vi "PTSAutoDailyEric.vi"() -> ()   [LabVIEW 2012]
uses:
  <vilib>/Utility/NIReport.llb/NI_report.lvclass
  <vilib>/addons/database/Connection.llb/DB Tools Open Connec (Path).vi
  <vilib>/addons/database/Connection.llb/Conn Execute.vi
  <vilib>/addons/database/Recordset.llb/Rec Fetch Recordset Data (R).vi
  <vilib>/addons/database/Recordset.llb/Rec Destroy - Connection.vi
  <vilib>/Utility/NIReport.llb/Append Text Table to Report (wrap).vi
  <vilib>/addons/database/_DB Variant To Data/Database Variant To Data.xnode
  <vilib>/addons/database/NI_Database_API.lvlib
  <vilib>/Utility/NIReport.llb/Excel/NI_Excel.lvclass
  <vilib>/addons/_office/NI_ReportGenerationToolkit.lvlib
panel:
  in  "Report Template":path=path "O:/Monitor/Report/PTSDailyReport.xls"
  in  "Table Control":string[][](table)
  out "error out 4":errorcluster
  out "error out":errorcluster
  out "appended array":string[](array[string])
  out "recordset data":variant[][](array[variant])
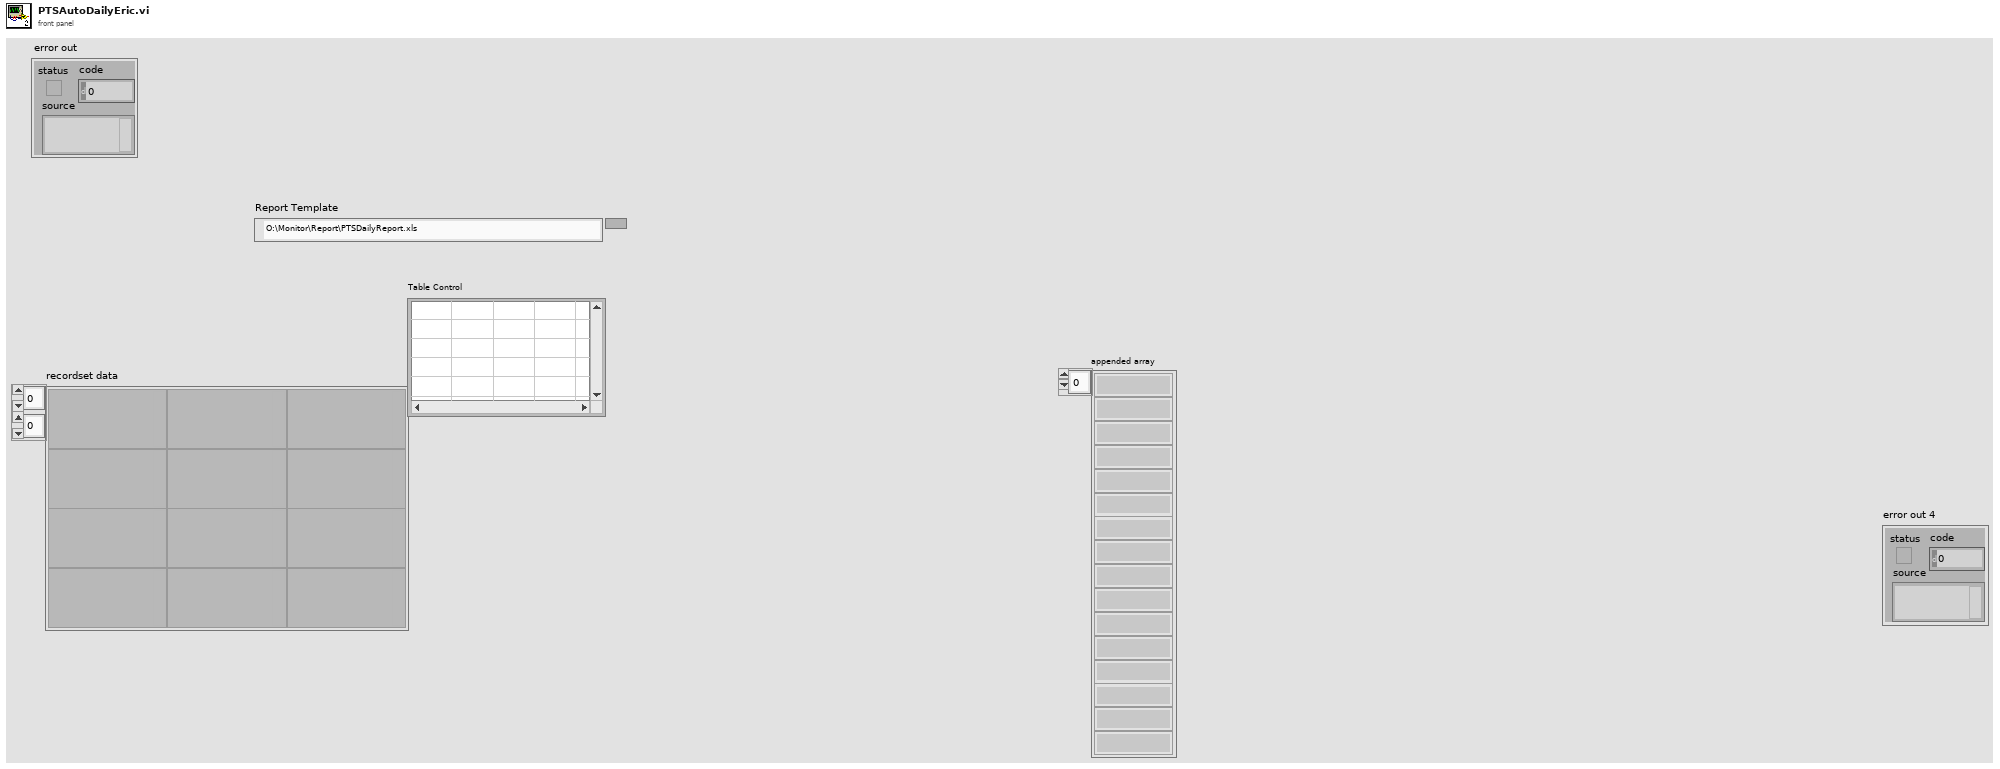
[diagram p1: front panel]
types:
  T1 = typedef "NI_Database_API.lvlib/Conn ObjectReference.ctl" = refnum<k1>
  T2 = typedef "NI_Database_API.lvlib/Rec ObjectReference.ctl" = refnum<k1>
  T3 = enum16{"Standard Report", "HTML", "Word", "Excel"}
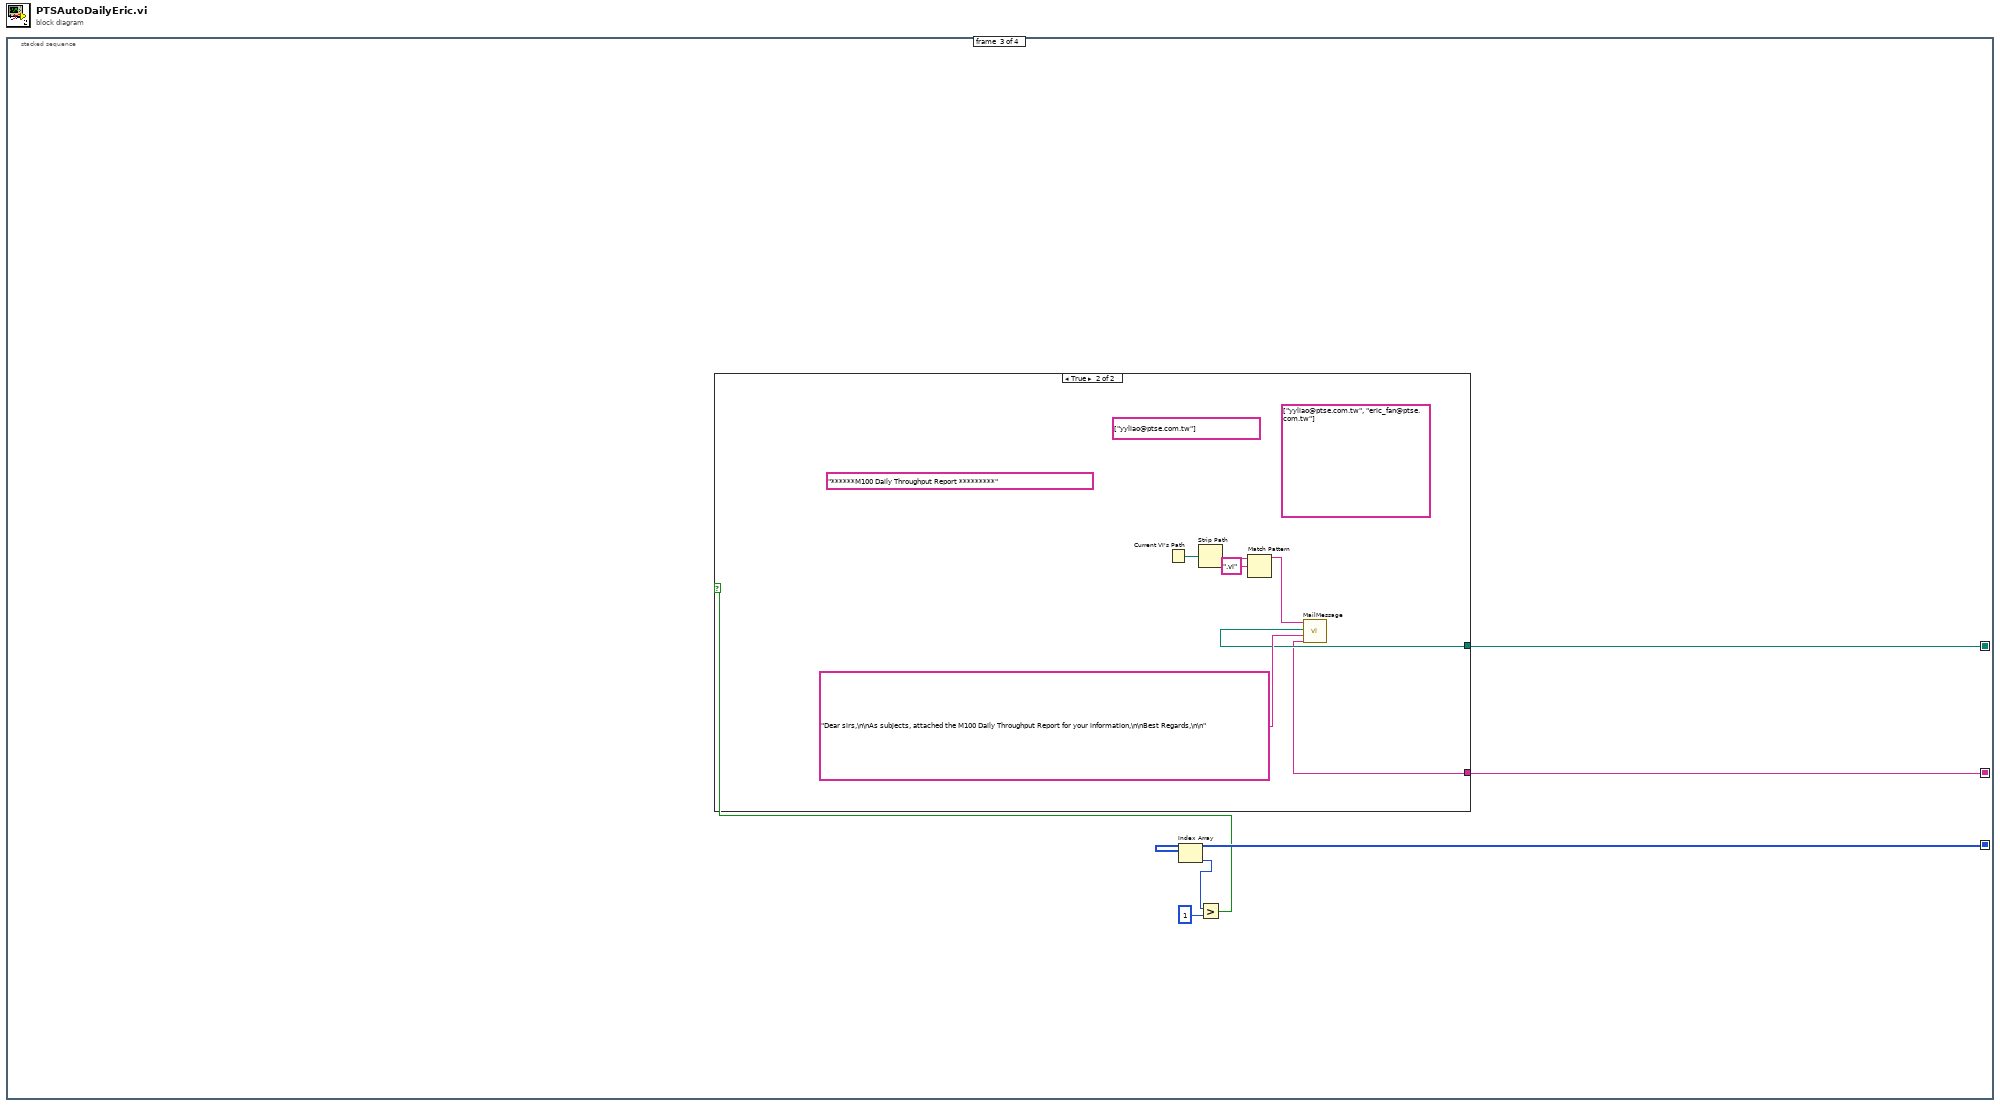
[diagram p0: block diagram]
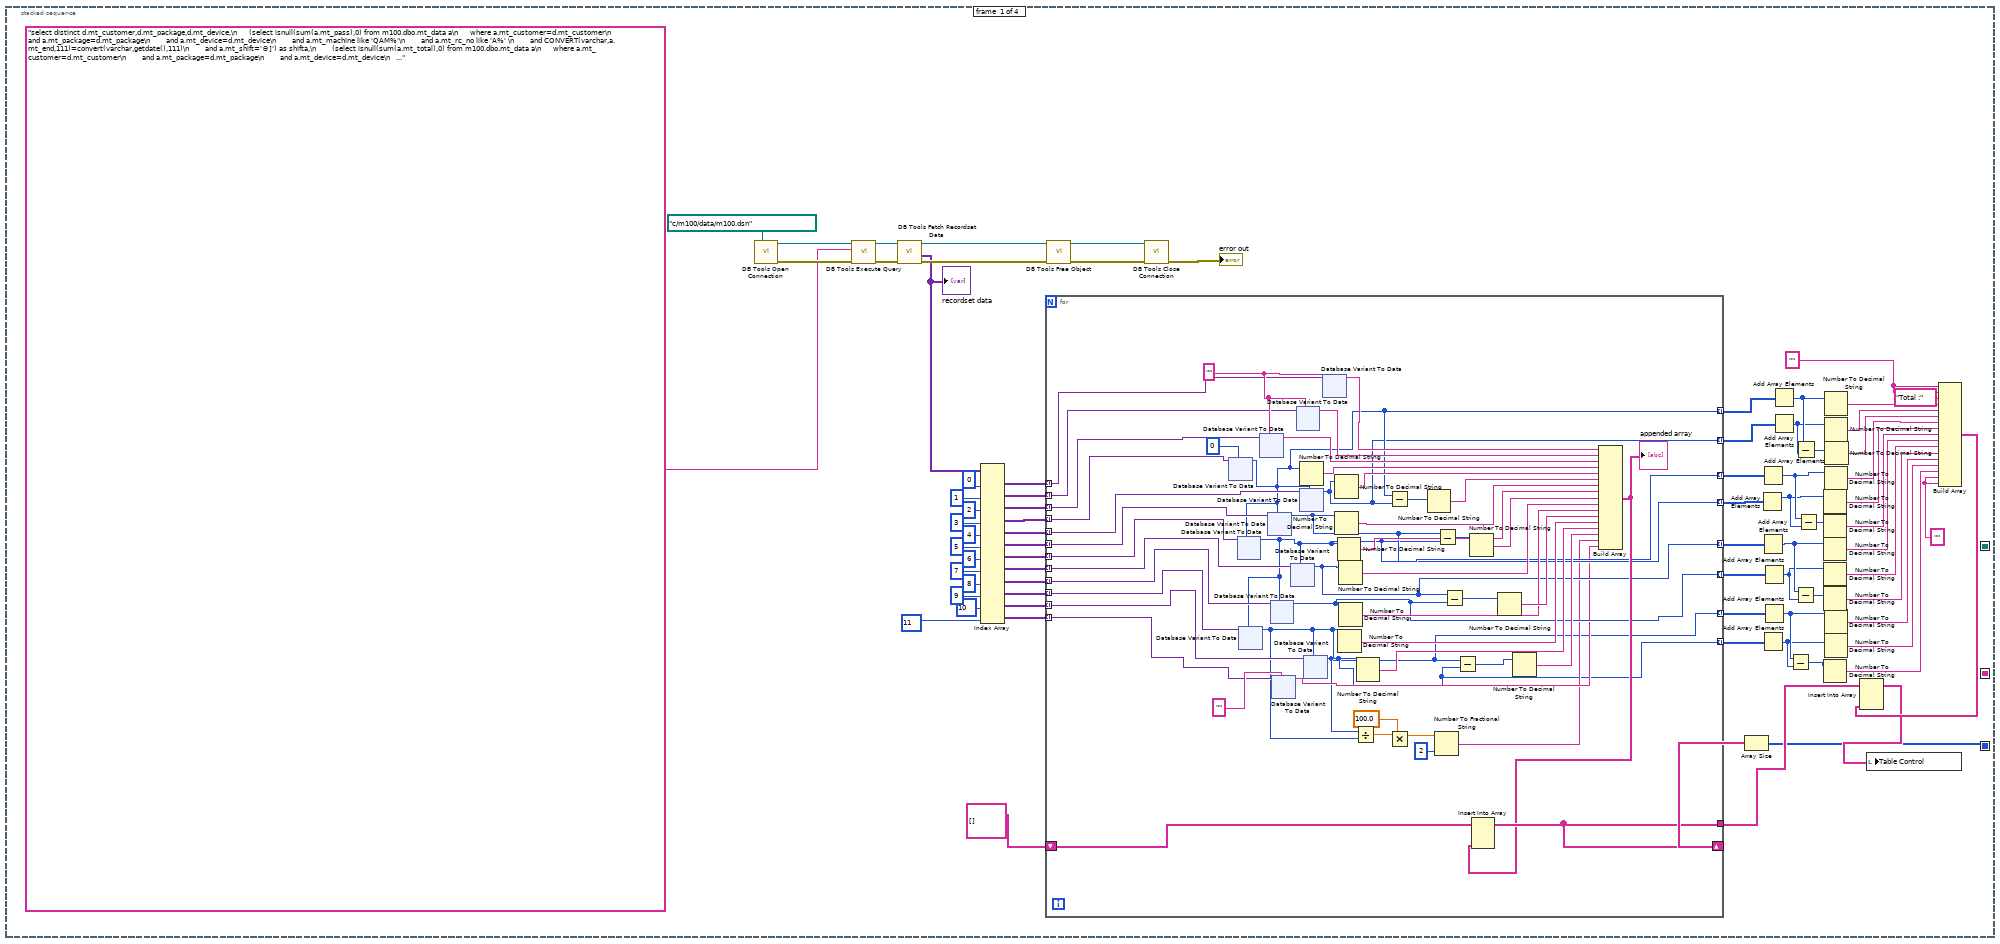
[diagram p2: hidden frame]
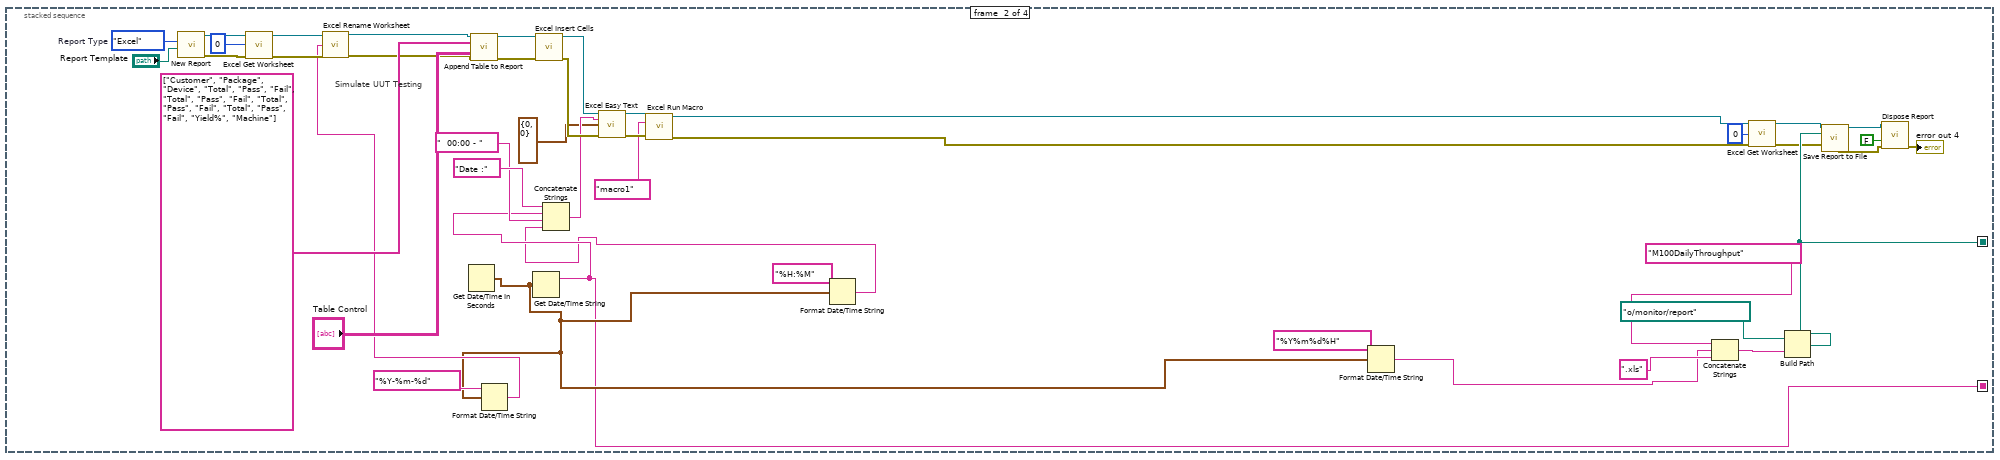
[diagram p3: hidden frame]
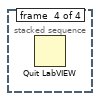
[diagram p5: hidden frame]
diagram:
  n1 = stacked-sequence {
    seq-local: [_ w541 _ _] -> [_ _ w562 _]
    seq-local: [_ w514 _ _] -> [_ _ w561 _]
    seq-local: [w2 _ _ _] -> [_ _ w560 _]
    frame #0 {
      w1 = ""
      w37 = ""
      n2 = call-poly <vilib>:"DB Tools Open Connection.vi"("connection information"=path "c:/m100/data/m100.dsn") -> ("error out"=w72:errorcluster, "connection reference"=w76:T1)  [unwired: 7 in]
      n3 = call-poly <vilib>:"DB Tools Execute Query.vi"("error in (no error)"=w72, "SQL query"="select distinct d.mt_customer,d.mt_package,d.mt_device,\n      (select isnull(sum(a.mt_pass),0) from m100.dbo.mt_data a\n      where a.mt_customer=d.mt_customer\n        and a.mt_package=d.mt_package\n        and a.mt_device=d.mt_device\n        and a.mt_machine like 'QAM%'\n        and a.mt_rc_no like 'A%' \n        and CONVERT(varchar,a.mt_end,111)=convert(varchar,getdate(),111)\n        and a.mt_shift='©]') as shifta,\n        (select isnull(sum(a.mt_total),0) from m100.dbo.mt_data a\n      where a.mt_customer=d.mt_customer\n        and a.mt_package=d.mt_package\n        and a.mt_device=d.mt_device\n        and a.mt_machine like 'QAM%'\n        and a.mt_rc_no like 'A%' \n        and CONVERT(varchar,a.mt_end,111)=convert(varchar,getdate(),111)\n        and a.mt_shift='©]') as shifta1,\n        (select isnull(sum(b.mt_pass),0) from m100.dbo.mt_data b\n      where b.mt_customer=d.mt_customer\n        and b.mt_package=d.mt_package\n       and b.mt_device=d.mt_device\n        and b.mt_machine like 'QAM%'\n        and b.mt_rc_no like 'A%' \n        and CONVERT(varchar,b.mt_end,111)=convert(varchar,getdate(),111)\n        and b.mt_shift='¦­') as shiftb,\n        (select isnull(sum(b.mt_total),0) from m100.dbo.mt_data b\n      where b.mt_customer=d.mt_customer\n        and b.mt_package=d.mt_package\n        and b.mt_device=d.mt_device\n        and b.mt_machine like 'QAM%'\n        and b.mt_rc_no like 'A%' \n        and CONVERT(varchar,b.mt_end,111)=convert(varchar,getdate(),111)\n        and b.mt_shift='¦­') as shiftb1,\n        (select isnull(sum(c.mt_pass),0) from m100.dbo.mt_data c\n      where c.mt_customer=d.mt_customer\n        and c.mt_package=d.mt_package\n        and c.mt_device=d.mt_device\n        and c.mt_machine like 'QAM%'\n        and c.mt_rc_no like 'A%' \n        and CONVERT(varchar,c.mt_end,111)=convert(varchar,getdate(),111)\n        and c.mt_shift='¤¤') as shiftc,\n        (select isnull(sum(c.mt_total),0) from m100.dbo.mt_data c\n      where c.mt_customer=d.mt_customer\n        and c.mt_package=d.mt_package\n        and c.mt_device=d.mt_device\n        and c.mt_machine like 'QAM%'\n        and c.mt_rc_no like 'A%' \n        and CONVERT(varchar,c.mt_end,111)=convert(varchar,getdate(),111)\n        and c.mt_shift='¤¤') as shiftc1,\n        SUM(mt_pass),SUM(mt_total),master.dbo.GetEntityNameFromDateToDate(d.mt_customer,d.mt_package,d.mt_device,CONVERT(varchar,GETDATE()-1,111),CONVERT(varchar,GETDATE(),111))\n  FROM [m100].[dbo].[mt_data] d\n  WHERE d.mt_machine like 'QAM%'\n    AND CONVERT(varchar,d.mt_end,111)=convert(varchar,getdate(),111)\n    and d.mt_pass > 0 and d.mt_rc_no like 'A%'\n      group by d.mt_customer,d.mt_package,d.mt_device", "connection reference"=w76) -> ("error out"=w71:errorcluster, "recordset reference"=w75:T2)  [unwired: 5 in]
      n4 = call-poly <vilib>:"DB Tools Fetch Recordset Data.vi"("error in (no error)"=w71, "recordset reference"=w75) -> ("error out"=w70:errorcluster, "recordset data"=w40:variant[][], "recordset reference out"=w74:T2)  [unwired: 3 in]
      "recordset data" <- w40
      n5 = Index Array(array=w40, index (col) #1=0 ("index (row)"), index (col) #2=1 ("index (col)"), index (col) #3=2 ("disabled index (col)"), index (col) #4=3 ("index (col)"), index (col) #5=4 ("index (col)"), index (col) #6=5 ("index (col)"), index (col) #7=6 ("index (col)"), index (col) #8=7 ("index (col)"), index (col) #9=8 ("index (col)"), index (col) #10=9 ("index (col)"), index (col) #11=10 ("index (col)"), index (col) #12=11 ("index (col)")) -> (element #1=w44:variant[], element #2=w43:variant[], element #3=w57:variant[], element #4=w56:variant[], element #5=w55:variant[], element #6=w54:variant[], element #7=w53:variant[], element #8=w52:variant[], element #9=w51:variant[], element #10=w50:variant[], element #11=w49:variant[], element #12=w48:variant[])  [unwired: 12 in]
      n6 = for {
        tunnel: w57 -> [w102] mode=indexing
        tunnel: w56 -> [w101] mode=indexing
        tunnel: w55 -> [w100] mode=indexing
        tunnel: w54 -> [w99] mode=indexing
        tunnel: w53 -> [w98] mode=indexing
        tunnel: w52 -> [w97] mode=indexing
        tunnel: w51 -> [w96] mode=indexing
        tunnel: w50 -> [w95] mode=indexing
        tunnel: w49 -> [w94] mode=indexing
        tunnel: w48 -> [w93] mode=indexing
        tunnel: [w128] -> w30
        shift-right: [w128] -> w46
        shift-left: string[][] [] ("array") -> [w127]
        tunnel: w44 -> [w104] mode=indexing
        tunnel: w43 -> [w103] mode=indexing
        tunnel: [w91] -> w39 mode=indexing
        tunnel: [w90] -> w38 mode=indexing
        tunnel: [w89] -> w28 mode=indexing
        tunnel: [w88] -> w27 mode=indexing
        tunnel: [w87] -> w19 mode=indexing
        tunnel: [w86] -> w18 mode=indexing
        tunnel: [w78] -> w11 mode=indexing
        tunnel: [w79] -> w10 mode=indexing
        w126 = ""
        n7 = xnode "Database Variant To Data"("database variant"=w101, "type"=0) -> ("data"=w91:i32)  [unwired: 1 in, 1 out]
        n8 = xnode "Database Variant To Data"("database variant"=w98, "type"=w91) -> ("data"=w88:i32)  [unwired: 1 in, 1 out]
        n9 = xnode "Database Variant To Data"("database variant"=w95, "type"=w88) -> ("data"=w78:i32)  [unwired: 1 in, 1 out]
        n10 = xnode "Database Variant To Data"("database variant"=w102, "type"=w126) -> ("data"=w110:string)  [unwired: 1 in, 1 out]
        n11 = xnode "Database Variant To Data"("database variant"=w99, "type"=w91) -> ("data"=w89:i32)  [unwired: 1 in, 1 out]
        n12 = xnode "Database Variant To Data"("database variant"=w96, "type"=w88) -> ("data"=w86:i32)  [unwired: 1 in, 1 out]
        n13 = xnode "Database Variant To Data"("database variant"=w93, "type"="") -> ("data"=w81:string)  [unwired: 1 in, 1 out]
        n14 = xnode "Database Variant To Data"("database variant"=w97, "type"=w88) -> ("data"=w87:i32)  [unwired: 1 in, 1 out]
        n15 = xnode "Database Variant To Data"("database variant"=w103, "type"=w126) -> ("data"=w107:string)  [unwired: 1 in, 1 out]
        n16 = Number To Decimal String(number=w91) -> (decimal integer string=w109:string)  [unwired: 1 in]
        n17 = xnode "Database Variant To Data"("database variant"=w100, "type"=w91) -> ("data"=w90:i32)  [unwired: 1 in, 1 out]
        n18 = xnode "Database Variant To Data"("database variant"=w94, "type"=w78) -> ("data"=w79:i32)  [unwired: 1 in, 1 out]
        n19 = xnode "Database Variant To Data"("database variant"=w104, "type"=w126) -> ("data"=w111:string)  [unwired: 1 in, 1 out]
        n20 = Number To Decimal String(number=w90) -> (decimal integer string=w108:string)  [unwired: 1 in]
        n21 = Number To Decimal String(number=w89) -> (decimal integer string=w124:string)  [unwired: 1 in]
        n22 = Number To Decimal String(number=w88) -> (decimal integer string=w123:string)  [unwired: 1 in]
        n23 = Number To Decimal String(number=w78) -> (decimal integer string=w118:string)  [unwired: 1 in]
        n24 = Number To Decimal String(number=w87) -> (decimal integer string=w114:string)  [unwired: 1 in]
        n25 = Number To Decimal String(number=w86) -> (decimal integer string=w115:string)  [unwired: 1 in]
        n26 = Divide(x=w79, y=w78) -> (x/y=w85:dbl)
        n27 = Number To Decimal String(number=w79) -> (decimal integer string=w119:string)  [unwired: 1 in]
        n28 = Subtract(x=w91, y=w90) -> (x-y=w106:i32)
        n29 = Multiply(x=w85, y=100.0) -> (x*y=w83:dbl)
        n30 = Number To Decimal String(number=w106) -> (decimal integer string=w105:string)  [unwired: 1 in]
        n31 = Number To Fractional String(number=w83, precision (6)=i16 2) -> (F-format string=w80:string)  [unwired: 2 in]
        n32 = Subtract(x=w89, y=w88) -> (x-y=w113:i32)
        n33 = Subtract(x=w87, y=w86) -> (x-y=w117:i32)
        n34 = Subtract(x=w78, y=w79) -> (x-y=w121:i32)
        n35 = Number To Decimal String(number=w113) -> (decimal integer string=w112:string)  [unwired: 1 in]
        n36 = Number To Decimal String(number=w117) -> (decimal integer string=w116:string)  [unwired: 1 in]
        n37 = Number To Decimal String(number=w121) -> (decimal integer string=w120:string)  [unwired: 1 in]
        n38 = Build Array(w111, w107, w110, w109, w108, w105, w124, w123, w112, w114, w115, w116, w118, w119, w120, w80, w81) -> (w92:string[])
        "appended array" <- w92
        n39 = Insert Into Array(array=w127, new element=w92) -> (w128:string[][])  [unwired: 2 in]
      }
      n40 = call-poly <vilib>:"DB Tools Free Object.vi"("error in (no error)"=w70, "recordset reference"=w74) -> ("error out"=w69:errorcluster, "connection reference"=w73:T1)  [unwired: 8 in]
      n41 = call <vilib>:"DB Tools Close Connection.vi"("error in (no error)"=w69, "connection reference"=w73) -> ("error out"=→"error out":errorcluster)  [unwired: 5 in]
      n42 = Array Size(array=w46) -> (size(s)=w2:i32[])
      n43 = Add Array Elements(numeric array=w27) -> (sum=w22:i32)
      n44 = Add Array Elements(numeric array=w28) -> (sum=w23:i32)
      n45 = Add Array Elements(numeric array=w19) -> (sum=w15:i32)
      n46 = Add Array Elements(numeric array=w10) -> (sum=w8:i32)
      n47 = Add Array Elements(numeric array=w18) -> (sum=w14:i32)
      n48 = Add Array Elements(numeric array=w11) -> (sum=w9:i32)
      n49 = Add Array Elements(numeric array=w39) -> (sum=w34:i32)
      n50 = Add Array Elements(numeric array=w38) -> (sum=w33:i32)
      n51 = Subtract(x=w9, y=w8) -> (x-y=w7:i32)
      n52 = Subtract(x=w15, y=w14) -> (x-y=w12:i32)
      n53 = Subtract(x=w34, y=w33) -> (x-y=w26:i32)
      n54 = Subtract(x=w23, y=w22) -> (x-y=w20:i32)
      n55 = Number To Decimal String(number=w22) -> (decimal integer string=w24:string)  [unwired: 1 in]
      n56 = Number To Decimal String(number=w20) -> (decimal integer string=w21:string)  [unwired: 1 in]
      n57 = Number To Decimal String(number=w15) -> (decimal integer string=w17:string)  [unwired: 1 in]
      n58 = Number To Decimal String(number=w14) -> (decimal integer string=w16:string)  [unwired: 1 in]
      n59 = Number To Decimal String(number=w12) -> (decimal integer string=w13:string)  [unwired: 1 in]
      n60 = Number To Decimal String(number=w7) -> (decimal integer string=w4:string)  [unwired: 1 in]
      n61 = Number To Decimal String(number=w34) -> (decimal integer string=w36:string)  [unwired: 1 in]
      n62 = Number To Decimal String(number=w33) -> (decimal integer string=w35:string)  [unwired: 1 in]
      n63 = Number To Decimal String(number=w23) -> (decimal integer string=w25:string)  [unwired: 1 in]
      n64 = Number To Decimal String(number=w9) -> (decimal integer string=w6:string)  [unwired: 1 in]
      n65 = Number To Decimal String(number=w8) -> (decimal integer string=w5:string)  [unwired: 1 in]
      n66 = Number To Decimal String(number=w26) -> (decimal integer string=w32:string)  [unwired: 1 in]
      n67 = Build Array(w37, w37, "Total :" ("element"), w36, w35, w32, w25, w24, w21, w17, w16, w13, w6, w5, w4, w1, w1) -> (w31:string[])
      n68 = Insert Into Array(array=w30, new element=w31) -> (w29:string[][])  [unwired: 2 in]
      n69 = local write "Table Control"(w29) -> ()
    }
    frame #1 {
      w556 = T3."Excel"  # Report Type
      # "Simulate UUT Testing"
      n70 = call <vilib>:"New Report.vi"("report type"=w556, "template (empty)"="Report Template") -> ("report out"=w552:refnum<class "NI_report.lvclass">, "error out"=w551:errorcluster)  [unwired: 12 in]
      n71 = call <vilib>:"Excel Get Worksheet.vi"("report in"=w552, "worksheet index (0)"=0, "error in (no error)"=w551) -> ("report out"=w530:refnum<class "NI_report.lvclass">, "error out"=w529:errorcluster)  [unwired: 11 in]
      n72 = Get Date/Time In Seconds() -> (seconds since 1Jan1904=w515:timestamp)
      n73 = Format Date/Time String(time format string (%c)="%Y-%m-%d", seconds (now)=w515) -> (date/time string=w525:string)  [unwired: 1 in]
      n74 = call <vilib>:"Excel Rename Worksheet.vi"("report in"=w530, "worksheet name (\"\")"=w525, "error in (no error)"=w529) -> ("report out"=w528:refnum<class "NI_report.lvclass">, "error out"=w527:errorcluster)  [unwired: 11 in]
      n75 = call-poly <vilib>:"Append Table to Report.vi"("report in"=w528, "column headers"=string[] ["Customer", "Package", "Device", "Total", "Pass", "Fail", "Total", "Pass", "Fail", "Total", "Pass", "Fail", "Total", "Pass", "Fail", "Yield%", "Machine"] ("row headers"), "text data"="Table Control", "error in (no error)"=w527) -> ("report out"=w554:refnum<class "NI_report.lvclass">, "error out"=w553:errorcluster)  [unwired: 8 in, 2 out]
      n76 = Get Date/Time String(seconds (now)=w515) -> (date string=w514:string)  [unwired: 2 in, 1 out]
      n77 = call <vilib>:"Excel Insert Cells.vi"("report in"=w554, "error in (no error)"=w553) -> ("report out"=w550:refnum<class "NI_report.lvclass">, "error out"=w549:errorcluster)  [unwired: 12 in]
      n78 = Format Date/Time String(time format string (%c)="%H:%M", seconds (now)=w515) -> (date/time string=w513:string)  [unwired: 1 in]
      n79 = Concatenate Strings("Date :" ("string"), w514, "  00:00 - " ("string"), w513) -> (w547:string)
      n80 = call <vilib>:"Excel Easy Text.vi"("report in"=w550, "text"=w547, "start (-1, -1)"=cluster{"row":i32, "column":i32} {"row"=0, "column"=0} ("end (-1, -1)"), "error in (no error)"=w549) -> ("report out"=w538:refnum<class "NI_report.lvclass">, "error out"=w537:errorcluster)  [unwired: 7 in, 3 out]
      n81 = call <vilib>:"Excel Run Macro.vi"("report in"=w538, "macro name"="macro1", "error in (no error)"=w537) -> ("report out"=w521:refnum<class "NI_report.lvclass">, "error out"=w519:errorcluster)  [unwired: 10 in, 1 out]
      n82 = Format Date/Time String(time format string (%c)="%Y%m%d%H", seconds (now)=w515) -> (date/time string=w517:string)  [unwired: 1 in]
      n83 = Concatenate Strings("M100DailyThroughput", w517, ".xls" ("string")) -> (w543:string)
      n84 = call <vilib>:"Excel Get Worksheet.vi"("report in"=w521, "worksheet index (0)"=0, "error in (no error)"=w519) -> ("report out"=w524:refnum<class "NI_report.lvclass">, "error out"=w523:errorcluster)  [unwired: 11 in]
      n85 = Build Path(base path=path "o:/monitor/report", name or relative path=w543) -> (appended path=w541:path)
      n86 = call-dynamic "Save Report to File.vi"("report in"=w524, "report file path"=w541, "error in (no error)"=w523) -> ("report out"=w532:refnum<class "NI_report.lvclass">, "error out"=w531:errorcluster)  [unwired: 11 in]
      n87 = call-dynamic "Dispose Report.vi"("report in"=w532, "save changes? (F)"=FALSE, "error in (no error)"=w531) -> ("error out"=→"error out 4":errorcluster)  [unwired: 12 in]
    }
    frame #2 {
      n88 = Index Array(array=w560) -> (element=w559:i32)  [unwired: 1 in]
      n89 = Greater?(x=w559, y=1) -> (0:w557:bool)
      n90 = case shown="True" w557 {
        tunnel: w562 -> [_ w564]
        tunnel: w561 -> [_ w563]
        frame False {
        }
        frame True {
          (unwired) string[] ["yyliao@ptse.com.tw", "eric_fan@ptse.com.tw"] ("recipients")
          (unwired) "******M100 Daily Throughput Report *********" ("subject ([No Subject])")
          (unwired) string[] ["yyliao@ptse.com.tw"] ("recipients")
          n91 = Current VI's Path() -> (path=w569:path)
          n92 = Strip Path(path=w569) -> (name=w568:string)  [unwired: 1 out]
          n93 = Match Pattern(string=w568, regular expression=".vi") -> (before substring=w566:string)  [unwired: 1 in, 3 out]
          n94 = call "MailMessage.vi"("AddSubject"=w563, "message"="Dear sirs,\n\nAs subjects, attached the M100 Daily Throughput Report for your information,\n\nBest Regards,\n\n", "file path"=w564, "program"=w566) -> ()  [unwired: 8 in]
        }
      }
    }
    frame #3 {
      n95 = Quit LabVIEW() -> ()  [unwired: 1 in]
    }
  }
